vi "英维克MB_api.vi"(6 "Slave ID":u8=1, 7 "STEP":enum16{"open", "read", "write", "close"}(ring)=enum."read", 8 "Error in":errorcluster caption="Error in (no error)", 9 "values":u16[](array[numeric]), 10 "quantity":u16, 11 "starting address":u16 format="%04xH") -> (0 "error out":errorcluster, 2 "MB session out":refnum<class "MB_Master.lvclass">, 3 "Registers":u16[](array[numeric]))   [LabVIEW 2016, in "环境动力监测库.lvlib" / "空调库.lvlib"]
uses:
  <vilib>/Plasmionique/MB Master/MB_Master/MB_Master.lvclass
  <vilib>/Plasmionique/MB Master/MB_Master_Serial/MB_Master_Serial.lvclass
  D:/Program Files (x86)/National Instruments/LabVIEW 2016/vi.lib/Plasmionique/MB Master/MB_Master/MB_Master.lvclass
  <vilib>/Plasmionique/MB Master/MB_Master_TCP/MB_Master_TCP.lvclass
  <vilib>/Plasmionique/MB Master/MB Master.lvlib
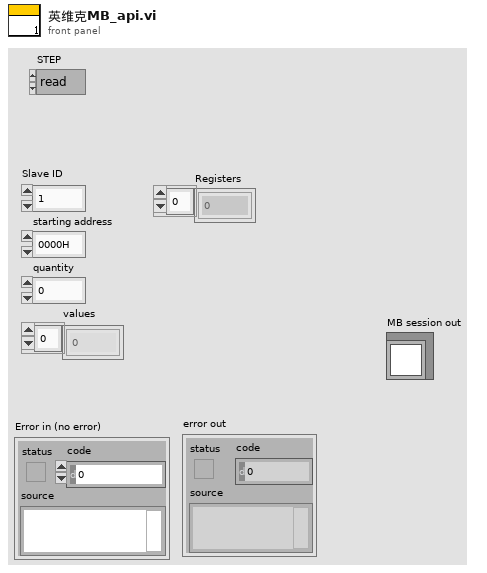
[diagram p1: front panel]
types:
  T1 = cluster{"baud rate (bps)":u32, "stop bits":u16, "parity":u16, "flow control":u16, "timeout":u32, "retries":i32}
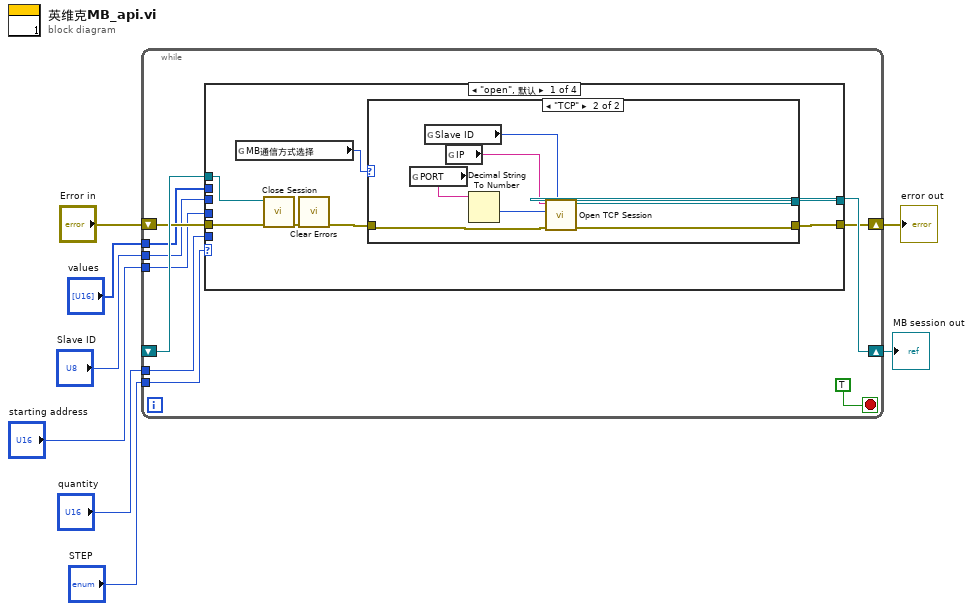
[diagram p0: block diagram]
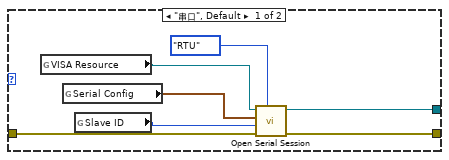
[diagram p2: hidden frame]
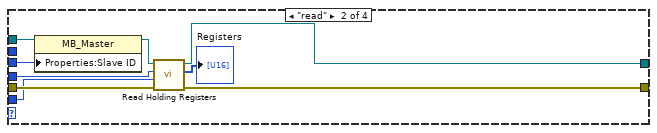
[diagram p3: hidden frame]
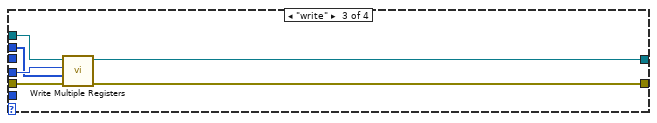
[diagram p4: hidden frame]
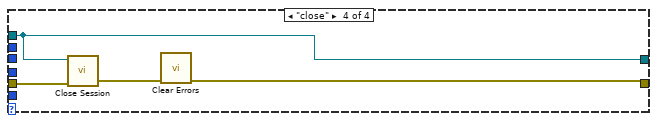
[diagram p5: hidden frame]
diagram:
  n1 = while {
    shift-right: [w10] -> w1
    shift-left: _ -> [w18]
    shift-right: [w9] -> w7
    shift-left: "Error in" -> [w17]
    tunnel: "Slave ID" -> [w16]
    tunnel: "starting address" -> [w15]
    tunnel: "quantity" -> [w14]
    tunnel: "STEP" -> [w13]
    tunnel: "values" -> [w12]
    stop <- TRUE stop-if-true
    n2 = case shown="\"open\", 默认" w13 {
      tunnel: w18 -> [w23 w41 w52 w57]
      tunnel: w17 -> [w22 w48 w54 w58]
      tunnel: [w24 w47 w51 w57] -> w10
      tunnel: [w25 w46 w53 w55] -> w9
      tunnel: w16 -> [_ w44 _ _]
      tunnel: w15 -> [_ w43 w50 _]
      tunnel: w14 -> [_ w42 _ _]
      tunnel: w12 -> [_ _ w49 _]
      frame "open", Default {
        n3 = global read "断电保存全局变量.vi" "MB通信方式选择"() -> (w19:enum16{"串口", "TCP"})
        n4 = call-dynamic "Close Session.vi"("error in (no error)"=w22, "MB session in"=w23) -> ("error out"=w21:errorcluster)  [unwired: 9 in]
        n5 = call <vilib>:"Clear Errors.vi"("error in (no error)"=w21) -> ("error out"=w20:errorcluster)  [unwired: 5 in, 1 out]
        n6 = case shown="\"TCP\"" w19 {
          tunnel: [w31 w37] -> w25
          tunnel: [w29 w36] -> w24
          tunnel: w20 -> [w30 w38]
          frame "串口", Default {
            n7 = global read "断电保存全局变量.vi" "VISA Resource"() -> (w28:refnum<visa-resource-name>)
            n8 = global read "断电保存全局变量.vi" "Serial Config"() -> (w27:T1)
            n9 = global read "断电保存全局变量.vi" "Slave ID"() -> (w26:u8)
            n10 = call <vilib>:"Open Serial Session.vi"("Mode (RTU)"=enum16{"RTU", "ASCII"}."RTU", "Error in"=w30, "Slave ID"=w26, "Serial Config"=w27, "VISA Resource"=w28) -> ("Error out"=w31:errorcluster, "MB_Serial session"=w29:refnum<class "MB_Master_Serial.lvclass">)  [unwired: 5 in]
          }
          frame "TCP" {
            n11 = global read "断电保存全局变量.vi" "PORT"() -> (w34:string)
            n12 = global read "断电保存全局变量.vi" "Slave ID"() -> (w33:u8)
            n13 = global read "断电保存全局变量.vi" "IP"() -> (w35:string)
            n14 = Decimal String To Number(string=w34) -> (number=w39:i32)  [unwired: 2 in, 1 out]
            n15 = call <vilib>:"Open TCP Session.vi"("Slave ID (255)"=w33, "error in (no error)"=w38, "Port (502)"=w39, "IP Address"=w35) -> ("error out"=w37:errorcluster, "MB_TCP session"=w36:refnum<class "MB_Master_TCP.lvclass">)  [unwired: 6 in]
          }
        }
      }
      frame "read" {
        n16 = property class="MB_Master"(reference=w41, "Properties:Slave ID"=w44) -> (reference out=w40:refnum<class "MB_Master.lvclass">)  [unwired: 1 in, 1 out]
        n17 = call <vilib>:"Read Holding Registers.vi"("error in (no error)"=w48, "quantity"=w42, "starting address"=w43, "MB session in"=w40) -> ("error out"=w46:errorcluster, "Registers"=→"Registers":u16[], "MB session out"=w47:refnum<class "MB_Master.lvclass">)  [unwired: 5 in]
      }
      frame "write" {
        n18 = call <vilib>:"Write Multiple Registers.vi"("error in (no error)"=w54, "values"=w49, "starting address"=w50, "MB session in"=w52) -> ("error out"=w53:errorcluster, "MB session out"=w51:refnum<class "MB_Master.lvclass">)  [unwired: 6 in]
      }
      frame "close" {
        n19 = call-dynamic "Close Session.vi"("error in (no error)"=w58, "MB session in"=w57) -> ("error out"=w56:errorcluster)  [unwired: 9 in]
        n20 = call <vilib>:"Clear Errors.vi"("error in (no error)"=w56) -> ("error out"=w55:errorcluster)  [unwired: 5 in, 1 out]
      }
    }
  }
  "error out" <- w7
  "MB session out" <- w1
